vi "Serial Comms Manager.vi"(7 "Action":T1, 10 "Serial Settings":T2={"baud rate"=9600, "data bits"=8, "parity"=enum."None", "stop bits"=10, "flow control"=0} {"flow control" items=["None"=0, "XON/XOFF"=1, "RTS/CTS"=2, "DTR/DSR"=4]; "stop bits" items=["1.0"=10, "1.5"=15, "2.0"=20]; "data bits" min=5 max=8 step=1; "baud rate" items=["75"=75, "110"=110, "134"=134, "150"=150, "300"=300, "600"=600, "1200"=1200, "1800"=1800, "2400"=2400, "4800"=4800, "7200"=7200, "9600"=9600, "14400"=14400, "19200"=19200, "28800"=28800, "38400"=38400, "56000"=56000, "57600"=57600, "115200"=115200, "128000"=128000, "230400"=230400]}, 11 "VISA Refnum in":refnum<visa-resource-name>) -> (2 "Success?":bool, 3 "VISA resource name out":refnum<visa-resource-name>)   [LabVIEW 2019]
uses:
  Serial - Settings.ctl
  Serial Connection States.ctl
  <vilib>/Utility/error.llb/DialogType.ctl
  <vilib>/Instr/_visa.llb/VISA Configure Serial Port (Instr).vi
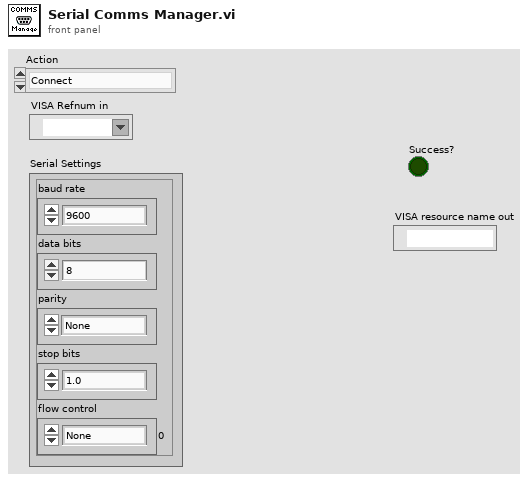
[diagram p1: front panel]
types:
  T1 = typedef "Serial Connection States.ctl" = enum16{"Connect", "Get Connection", "Disconnect"}
  T2 = typedef "Serial - Settings.ctl" = cluster{"baud rate":u32, "data bits":u16, "parity":enum16{"None", "Odd", "Even", "Mark", "Space"}, "stop bits":u16, "flow control":u16}
  T3 = typedef "DialogType.ctl" = u16
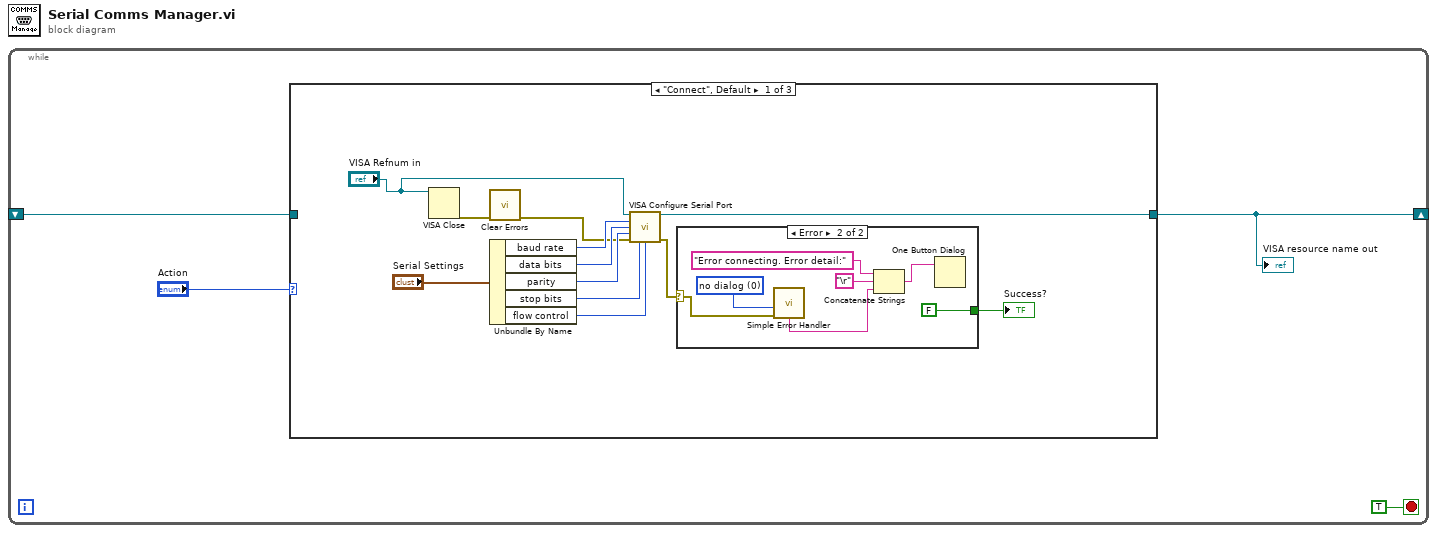
[diagram p0: block diagram]
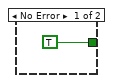
[diagram p2: hidden frame]
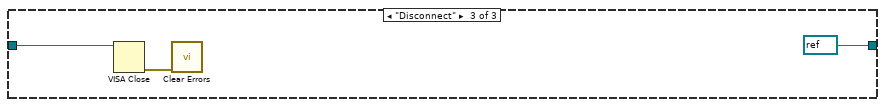
[diagram p4: hidden frame]
diagram:
  n1 = while {
    shift-right: [w1] -> _
    shift-left: _ -> [w3]
    stop <- TRUE stop-if-true
    n2 = case shown="\"Connect\", Default" "Action" {
      tunnel: [w9 w25 refnum<visa-resource-name> refnum ("VISA resource name out")] -> w1
      tunnel: w3 -> [_ w25 w28]
      frame "Connect", Default {
        n3 = VISA Close(VISA resource name="VISA Refnum in") -> (error out=w6:errorcluster)  [unwired: 1 in]
        n4 = call <vilib>:"Clear Errors.vi"("error in (no error)"=w6) -> ("error out"=w5:errorcluster)  [unwired: 5 in, 1 out]
        n5 = Unbundle By Name("Serial Settings") -> ("baud rate"=w12:u32, "data bits"=w13:u16, "parity"=w14:enum16{"None", "Odd", "Even", "Mark", "Space"}, "stop bits"=w10:u16, "flow control"=w15:u16)
        n6 = call-poly "VISA Configure Serial Port"("VISA resource name"="VISA Refnum in", "baud rate (9600)"=w12, "data bits (8)"=w13, "parity (0:none)"=w14, "error in (no error)"=w5, "stop bits (10: 1 bit)"=w10, "flow control (0:none)"=w15) -> ("VISA resource name out"=w9:refnum<visa-resource-name>, "error out"=w16:errorcluster)  [unwired: 2 in, 5 out]
        n7 = case shown="Error" w16 {
          selector: w16 -> [_ w19]
          tunnel: [TRUE FALSE] -> w8
          frame No Error {
          }
          frame Error {
            w20 = T3 0 items=["no dialog", "OK message", "continue or stop message", "OK message + warnings", "continue/stop + warnings"] ("type of dialog (OK msg:1)")
            n8 = call <vilib>:"Simple Error Handler.vi"("type of dialog (OK msg:1)"=w20, "error in (no error)"=w19) -> ("message"=w18:string)  [unwired: 3 in, 4 out]
            n9 = Concatenate Strings("Error connecting. Error detail:" ("message"), "\r", w18) -> (w22:string)
            n10 = One Button Dialog(message=w22) -> ()  [unwired: 1 in, 1 out]
          }
        }
        "Success?" <- w8
      }
      frame "Get Connection" {
      }
      frame "Disconnect" {
        n11 = VISA Close(VISA resource name=w28) -> (error out=w26:errorcluster)  [unwired: 1 in]
        n12 = call <vilib>:"Clear Errors.vi"("error in (no error)"=w26) -> ()  [unwired: 5 in, 2 out]
      }
    }
    "VISA resource name out" <- w1
  }
